vi "UpperMidbrain.vi"(5 "Boat Heading":i8, 6 "tweak":T1, 7 "WhatAroundMeMap? 2":cluster{"T":dbl, "Range":dbl, "Bearing":dbl}[](array[cluster]), 8 "SOFT E-STOP":bool, 9 "behavior weights":i8[](array[numeric])=[0, 1, 0], 10 "ir distance":i32, 11 "Forebrain to Midbrain":cluster{"t":i16, "RudderAngle":i16}) -> (3 "string":string)   [LabVIEW 2012]
uses:
  NINJA Code/Tugboat/Robo_Programs/behaviorOutput_t.ctl
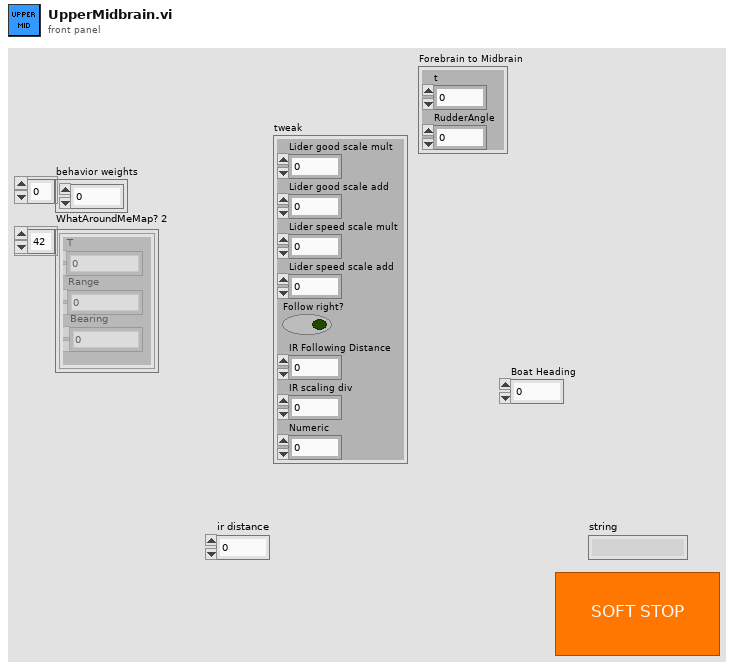
[diagram p1: front panel]
types:
  T1 = cluster{"Lider good scale mult":dbl, "Lider good scale add":dbl, "Lider speed scale mult":dbl, "Lider speed scale add":dbl, "Follow right?":bool, "IR Following Distance":i32, "IR scaling div":dbl, "Numeric":dbl}
  T2 = typedef "behaviorOutput_t.ctl" = cluster{"Goodness":i8[], "Velocity":i8[], "Weight":i8}
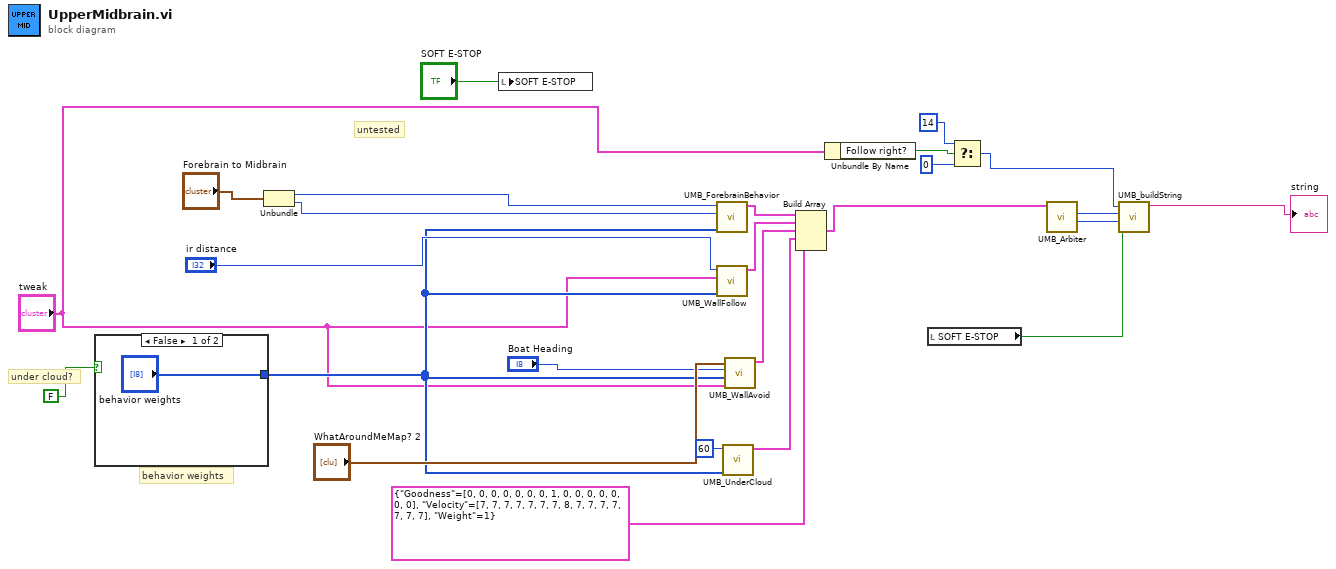
[diagram p0: block diagram]
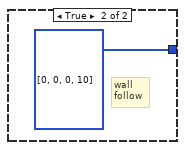
[diagram p2: hidden frame]
diagram:
  # "under cloud?"
  # "behavior weights"
  # "untested"
  n1 = case shown="False" FALSE {
    tunnel: ["behavior weights" i8[] [0, 0, 0, 10] ("behavior weights 2")] -> w11
    frame False {
    }
    frame True {
      # "wall\nfollow"
    }
  }
  n2 = Unbundle("Forebrain to Midbrain") -> ("t"=w1:i16, "RudderAngle"=w2:i16)
  n3 = local write "SOFT E-STOP"("SOFT E-STOP") -> ()
  n4 = call "UMB_ForebrainBehavior.vi"("behavior weights"=w11, "Desired Velocity"=w2, "Desired Heading"=w1) -> ("Behavior Output"=w19:T2)  [unwired: 8 in]
  n5 = call "UMB_WallFollow.vi"("behavior weights"=w11, "tweak cluster"="tweak", "ir distance"="ir distance") -> ("Behavior Output"=w17:T2)  [unwired: 8 in]
  n6 = call "UMB_UnderCloud.vi"("behavior weights"=w11, "Boat Heading"=60) -> ("Behavior Output"=w13:T2)  [unwired: 9 in]
  n7 = call "UMB_WallAvoid.vi"("tweak cluster"="tweak", "behavior weights"=w11, "Boat Heading"="Boat Heading", "WhatAroundMeMap?"="WhatAroundMeMap? 2") -> ("Behavior Output"=w16:T2)  [unwired: 7 in]
  n8 = Build Array(w19, w17, w16, w13, T2 {"Goodness"=[0, 0, 0, 0, 0, 0, 0, 1, 0, 0, 0, 0, 0, 0, 0], "Velocity"=[7, 7, 7, 7, 7, 7, 7, 8, 7, 7, 7, 7, 7, 7, 7], "Weight"=1} ("Behavior Output")) -> (w20:T2[])
  n9 = Unbundle By Name("tweak") -> ("Follow right?"=w6:bool)
  n10 = local read "SOFT E-STOP"() -> (w24:bool)
  n11 = Select(t=i8 14, s=w6, f=i8 0) -> (s? t:f=w7:i8)
  n12 = call "UMB_Arbiter.vi"("Behavior Data"=w20) -> ("prop"=w21:i8, "rudder"=w22:i32)  [unwired: 9 in]
  n13 = call "UMB_buildString.vi"("soft e-stop"=w24, "Prop"=w21, "Rudder"=w22, "IR Servo"=w7) -> ("string"=→"string":string)  [unwired: 7 in]
